vi "HMI-Malicious-DE.vi"() -> ()   [LabVIEW 2018]
uses:
  <vilib>/Platform/TimedLoop/XDataNode/timing_clust.ctl
  <vilib>/Platform/TimedLoop/XDataNode/nitl_modes.ctl
  <vilib>/Platform/TimedLoop/XDataNode/wakeup.ctl
  <vilib>/Platform/TimedLoop/XDataNode/XDataNode.xnode
  <vilib>/Platform/TimedLoop/XDataNode/XDNodeRunTimeDep.lvlib
panel:
  out "TX Loop Iterations":i32
  out "Data sent":dbl
  out "Data generated":dbl
  out "error out":errorcluster
  in  "IP address":string="192.168.0.5"
  in  "Receiver Port number":u16=52557
  in  "error in (no error)":errorcluster
  in  "Transmitter port number":u16=12345
  out "Malicious Loop Iterations":i32
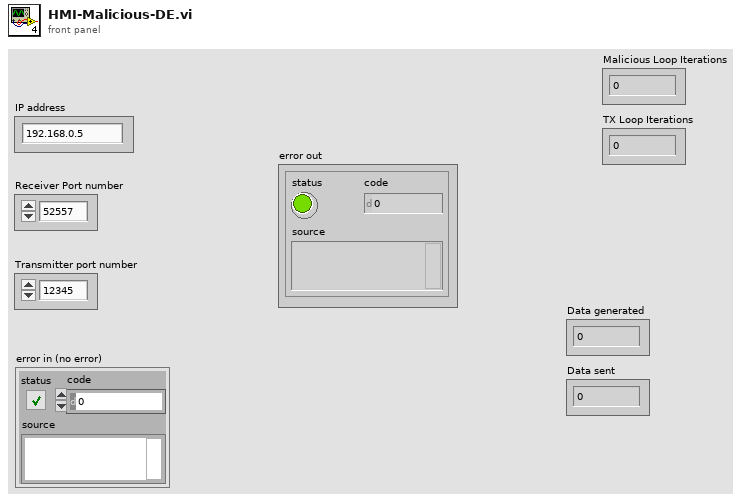
[diagram p1: front panel]
types:
  T1 = typedef "XDNodeRunTimeDep.lvlib/timing_clust.ctl" = cluster{"Expected End [f-1]":u64, "Actual End [f-1]":u64, "Finished Late? [f-1]":bool, "Expected End [i-1]":u64, "Actual End [i-1]":u64, "Finished Late? [i-1]":bool, "Expected Start [i]":u64, "Actual Start [i]":u64, "Expected Start [f]":u64, "Actual Start [f]":u64, "Source Name":string, "Structure Name":string, "Period":i64, "Deadline":i64, "Offset":i64, "Start":i64, "Priority":i32, "Timeout":i32, "Mode":T2, "Wakeup Reason":T3, "Error":errorcluster, "Source Type":string, "Secondary Source Type":string, "Global End Time":u64, "Global Start Time":u64, "Frame Duration":u64, "Iteration Duration":u64, "Assigned CPU":i32, "I/O Scan Engine Mode":u32}
  T2 = typedef "XDNodeRunTimeDep.lvlib/nitl_modes.ctl" = enum32{"No Change", "Process missed periods, maintain original phase", "Discard missed periods, maintain original phase", "Process missed periods, ignore original phase", "Discard missed periods, ignore original phase"}
  T3 = typedef "XDNodeRunTimeDep.lvlib/wakeup.ctl" = enum32{"Normal", "Aborted", "Asynchronous wakeup", "Timing source error", "Timed loop error", "Timeout"}
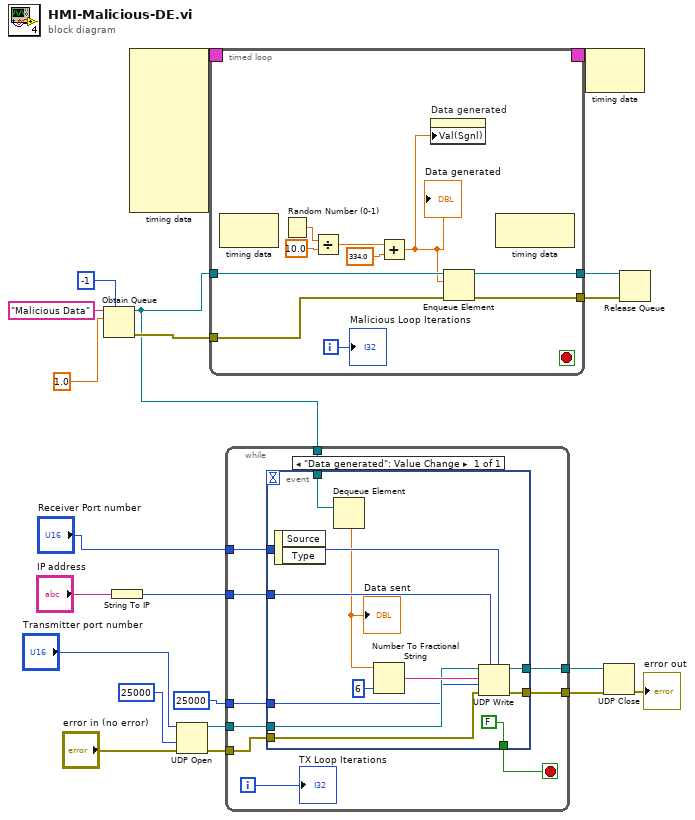
[diagram p0: block diagram]
diagram:
  n1 = Obtain Queue(max queue size (-1, unlimited)=-1, name (unnamed)="Malicious Data", element data type=1.0) -> (queue out=w1:refnum<queue>, error out=w5:errorcluster)  [unwired: 2 in, 1 out]
  n2 = String To IP(1:"IP address") -> (0:w15:u32)
  n3 = node-c288() -> (w21:T1)  [unwired: 9 in]
  n4 = UDP Open(8:"error in (no error)", 9:25000 ("timeout ms (25000)"), 11:"Transmitter port number") -> (port=w13:refnum<k16>, 0:w11:errorcluster)  [unwired: 2 in, 1 out]
  n5 = timed-loop {
    timing: w21 -> [_]
    timing-out: [_] -> w20
    tunnel: w1 -> [w26]
    tunnel: w5 -> [w25]
    tunnel: [w24] -> w4
    tunnel: [w23] -> w3
    i -> [w27]
    stop <- _ stop-if-true
    n6 = node-c288() -> ()  [unwired: 1 in, 1 out]
    n7 = Random Number (0-1)() -> (number: 0 to 1=w29:dbl)
    n8 = Divide(x=w29, y=10.0) -> (x/y=w28:dbl)
    n9 = Add(x=w28, y=334.0) -> (x+y=w22:dbl)
    "Data generated" <- w22
    n10 = property on="Data generated" class="DigNum (strict)"("Val(Sgnl)"=w22) -> ()  [unwired: 2 in, 2 out]
    n11 = Enqueue Element(queue=w26, element=w22, error in (no error)=w25) -> (queue out=w23:refnum<queue>, error out=w24:errorcluster)  [unwired: 1 in, 1 out]
    n12 = node-c288() -> ()  [unwired: 1 in, 1 out]
    "Malicious Loop Iterations" <- w27
  }
  n13 = while {
    tunnel: w15 -> [w43]
    tunnel: "Receiver Port number" -> [w42]
    tunnel: w13 -> [w41]
    tunnel: 25000 ("timeout ms (25000)") -> [w40]
    tunnel: w11 -> [w39]
    tunnel: [w38] -> w10
    tunnel: [w37] -> w9
    tunnel: w1 -> [w36]
    i -> [w35]
    stop <- w34 stop-if-true
    n14 = event shown="[0] \"Data generated\": Value Change" {
      selector: _ -> [_]
      dyn-events: _ -> [_]
      timeout: _ -> [_]
      tunnel: w43 -> [w53]
      tunnel: w42 -> [w52]
      tunnel: w41 -> [w51]
      tunnel: w40 -> [w50]
      tunnel: w39 -> [w49]
      tunnel: [w48] -> w38
      tunnel: [w47] -> w37
      tunnel: w36 -> [w46]
      tunnel: [FALSE] -> w34
      event "Data generated": Value Change {
        n15 = event-data() -> ()  [unwired: 1 in, 2 out]
        n16 = Dequeue Element(queue=w46) -> (element=w45:dbl)  [unwired: 2 in, 3 out]
        "Data sent" <- w45
        n17 = Number To Fractional String(number=w45, precision (6)=i16 6) -> (F-format string=w54:string)  [unwired: 2 in]
        n18 = UDP Write(address=w53, port or service name=w52, connection ID=w51, data in=w54, 8:w49, 9:w50) -> (error out=w47:errorcluster, 3:w48:refnum<k16>)
      }
    }
    "TX Loop Iterations" <- w35
  }
  n19 = node-c288(w20) -> ()  [unwired: 1 out]
  n20 = UDP Close(connection ID=w10, 8:w9) -> (error out=→"error out":errorcluster)  [unwired: 1 out]
  n21 = Release Queue(queue=w3, error in (no error)=w4) -> ()  [unwired: 1 in, 3 out]
